vi "Monitor FIFO Health.vi"(9 "stream.reset health monitor 0":bool, 10 "samples in fifo":u32) -> (0 "stream.min samples ready 0":u32, 1 "stream.max samples ready 0":u32, 2 "stream.num samples ready 0":u32)   [LabVIEW 2015, in "niInstr Streaming v1 FPGA.lvlib"]
doc: "Monitor FIFO Health is used to enable applications to keep track of various parameters of a FIFO under control. It is an optional VI, which is often most useful in helping to diagnose problems with throughput. A user may also use this VI to allow the host to wait for the FIFO to be full enough or empty enough to begin a transfer. This is commonly called \"priming the FIFO\" - ensuring that data is available to use before one starts a stream. A user who would prefer the FPGA to manage waiting for the FIFO to be primed may prefer to use the VI <b>Monitor Minimum Samples Ready</b> for the task.\n\nAll terminals with a number suffix are intended to be connected to the host by controls and indicators. The number allows the host to resolve different stream numbers from the host interface. Note: some terminals are optional.\n\nThis VI is commonly used in conjunction with the host VIs <b>Wait for Samples Ready</b> or <b>Get Stream Samples Ready</b>, which inspect the value in <b>stream.num samples ready N</b>.\n\n<b>samples in fifo</b>\n\nA user should connect the output of the FPGA FIFO Method \"Get Number of Elements to Read\" or \"Get Number of Elements to Write\" for the FIFO that will be monitored.\n\n<b>stream.reset health monitor N</b>\n\nConnect a control to this VI to allow the host to clear the state of the monitor. This will clear the memory of the outputs <b>stream.max samples ready</b> and <b>stream.min samples ready</b>\n\n<b>stream.num samples ready N</b> reflects the current value reported to the <b>samples in fifo</b> terminal.\n\n<b>stream.max samples ready N</b> and <b>stream.min samples ready N</b> reflect the highest value and the lowest value reported to the <b>samples in fifo</b> terminal since the last reset."
uses:
  <instrlib>/_niInstr/Streaming/v1/FPGA/niInstr Streaming v1 FPGA.lvlib
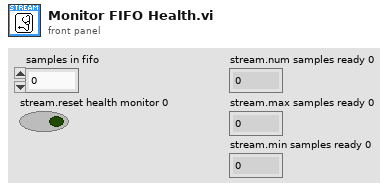
[diagram p1: front panel]
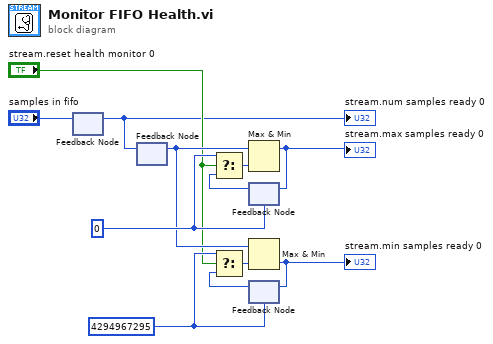
[diagram p0: block diagram]
diagram:
  w5 = u32 4294967295
  w10 = u32 0
  n1 = feedback #1() -> (w1:u32)  [unwired: 1 in]
  "stream.num samples ready 0" <- w1
  n2 = feedback-in #1("samples in fifo") -> ()
  n3 = feedback-in #2(w1) -> ()
  n4 = feedback #2() -> (w6:u32)  [unwired: 1 in]
  n5 = feedback #3(w10) -> (w9:u32)
  n6 = Select(t=w10, s="stream.reset health monitor 0", f=w9) -> (s? t:f=w11:u32)
  n7 = Max & Min(x=w6, y=w11) -> (max(x,y)=w12:u32)  [unwired: 1 out]
  "stream.max samples ready 0" <- w12
  n8 = feedback-in #3(w12) -> ()
  n9 = feedback #4(w5) -> (w8:u32)
  n10 = Select(t=w5, s="stream.reset health monitor 0", f=w8) -> (s? t:f=w7:u32)
  n11 = Max & Min(x=w6, y=w7) -> (min(x,y)=w3:u32)  [unwired: 1 out]
  "stream.min samples ready 0" <- w3
  n12 = feedback-in #4(w3) -> ()
